vi "Add EDS.vi"(9 "EDS":refnum<class "EDS.lvclass">, 10 "File Path":path, 11 "UI Actor in":refnum<class "UI Actor.lvclass">) -> (3 "UI Actor out":refnum<class "UI Actor.lvclass">)   [LabVIEW 2024, in "UI Actor.lvlib" / "UI Actor.lvclass"]
uses:
  UI Actor.lvclass
  UI Actor.lvclass/UI Actor.ctl
  Core/EDS/EDS.lvclass
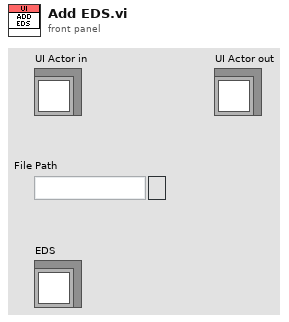
[diagram p1: front panel]
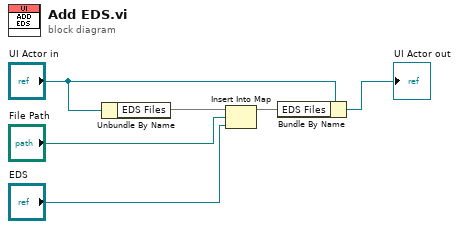
[diagram p0: block diagram]
diagram:
  n1 = Unbundle By Name("UI Actor in") -> ("EDS Files"=w4:map{path, refnum<class "EDS.lvclass">})
  n2 = Insert Into Map(map in=w4, key="File Path", value="EDS") -> (map out=w1:map{path, refnum<class "EDS.lvclass">})  [unwired: 2 out]
  n3 = Bundle By Name(cluster="UI Actor in", "EDS Files"=w1) -> (→"UI Actor out":refnum<class "UI Actor.lvclass">)
